vi "set_remote-interface-mode.vi"(8 "error in (no error)":errorcluster, 10 "mode":u16(ring) items=["local", "remote", "remot with lock-out"], 11 "Pfeiffer MultiGauge TPG256 in":refnum<class "Pfeiffer MultiGauge TPG256.lvclass">) -> (0 "error out":errorcluster, 3 "Pfeiffer MultiGauge TPG256 out":refnum<class "Pfeiffer MultiGauge TPG256.lvclass">)   [LabVIEW 2018, in "Pfeiffer MultiGauge TPG256.lvclass"]
doc: "sets the remote interface of the actual instrument.\nMode=1 (local), 2 (remote), 3 (remote with lockout)"
uses:
  Pfeiffer MultiGauge TPG256.lvclass
  instrument.lvclass
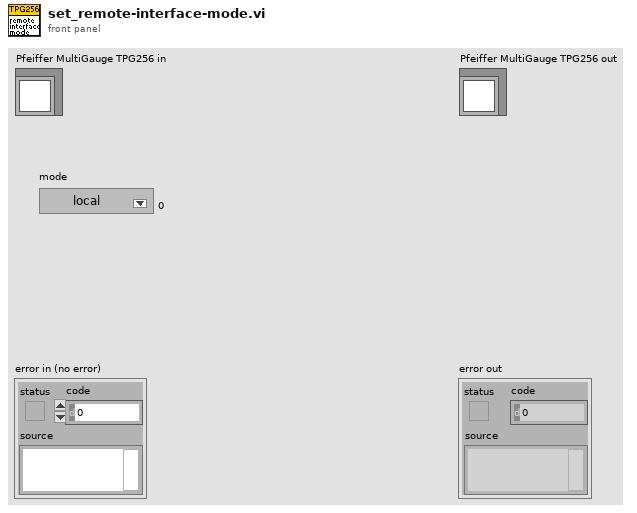
[diagram p1: front panel]
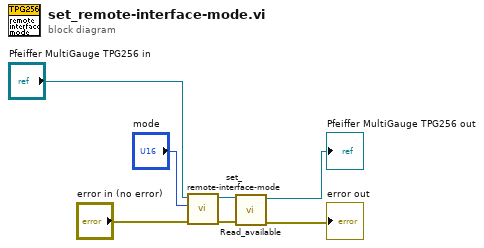
[diagram p0: block diagram]
diagram:
  n1 = call-parent "set_remote-interface-mode.vi"("error in (no error)"="error in (no error)", "mode"="mode", "instrument in"="Pfeiffer MultiGauge TPG256 in") -> ("error out"=w3:errorcluster, "instrument out"=w4:refnum<class "Pfeiffer MultiGauge TPG256.lvclass">)  [unwired: 7 in]
  n2 = call-dynamic "Read_available.vi"("error in (no error)"=w3, "instrument in"=w4) -> ("error out"=→"error out":errorcluster, "instrument out"=→"Pfeiffer MultiGauge TPG256 out":refnum<class "Pfeiffer MultiGauge TPG256.lvclass">)  [unwired: 7 in, 1 out]
